vi "Teleop.vi"(10 "Match Info out":T2={"Autonomous Elapsed Seconds"=0.0, "TeleOp Elapsed Seconds"=0.0, "Disabled Elapsed Seconds"=0.0, "Visited Autonomous"=FALSE, "Visited TeleOp"=FALSE, "Visited Disabled"=FALSE, "Autonomous Settings"={"Autonomous Style"=enum."Independent", "VI Refnum"=refnum}}, 11 "Call Context":T3) -> ()   [LabVIEW 2015]
doc: "This VI is called for each TeleOp packet received from the DS where the robot is not disabled. It is often used to read from the joysticks and update I/O or to update setpoints for timed control loops. It should complete and return within 20 milliseconds or it may miss DS packets."
uses:
  Robot Global Data.vi
  <vilib>/Rock Robotics/WPI/RobotDrive/WPI_RobotDriveMecanumDrive_Cartesian.vi
  <vilib>/addons/control/pid/NI_PID_pid.lvlib
  <vilib>/addons/control/pid/pid.llb/PID (DBL).vi
  <vilib>/Rock Robotics/WPI/DriverStation/WPI_DriverStationDerivedRobotMode.ctl
  <vilib>/Rock Robotics/WPI/DriverStation/WPI_DriverStationMatch Info.ctl
panel:
  out "Gyro":T1(graph)
  out "Rotation Input":dbl(graph)
  out "Numeric 1":dbl(slide) scale=0.0..100.0
  out "Boolean 2":bool
  out "Boolean 1":bool
  in  "Match Info":T2={"Autonomous Elapsed Seconds"=0.0, "TeleOp Elapsed Seconds"=0.0, "Disabled Elapsed Seconds"=0.0, "Visited Autonomous"=FALSE, "Visited TeleOp"=FALSE, "Visited Disabled"=FALSE, "Autonomous Settings"={"Autonomous Style"=enum."Independent", "VI Refnum"=refnum}}
  in  "Call Context 2":T3
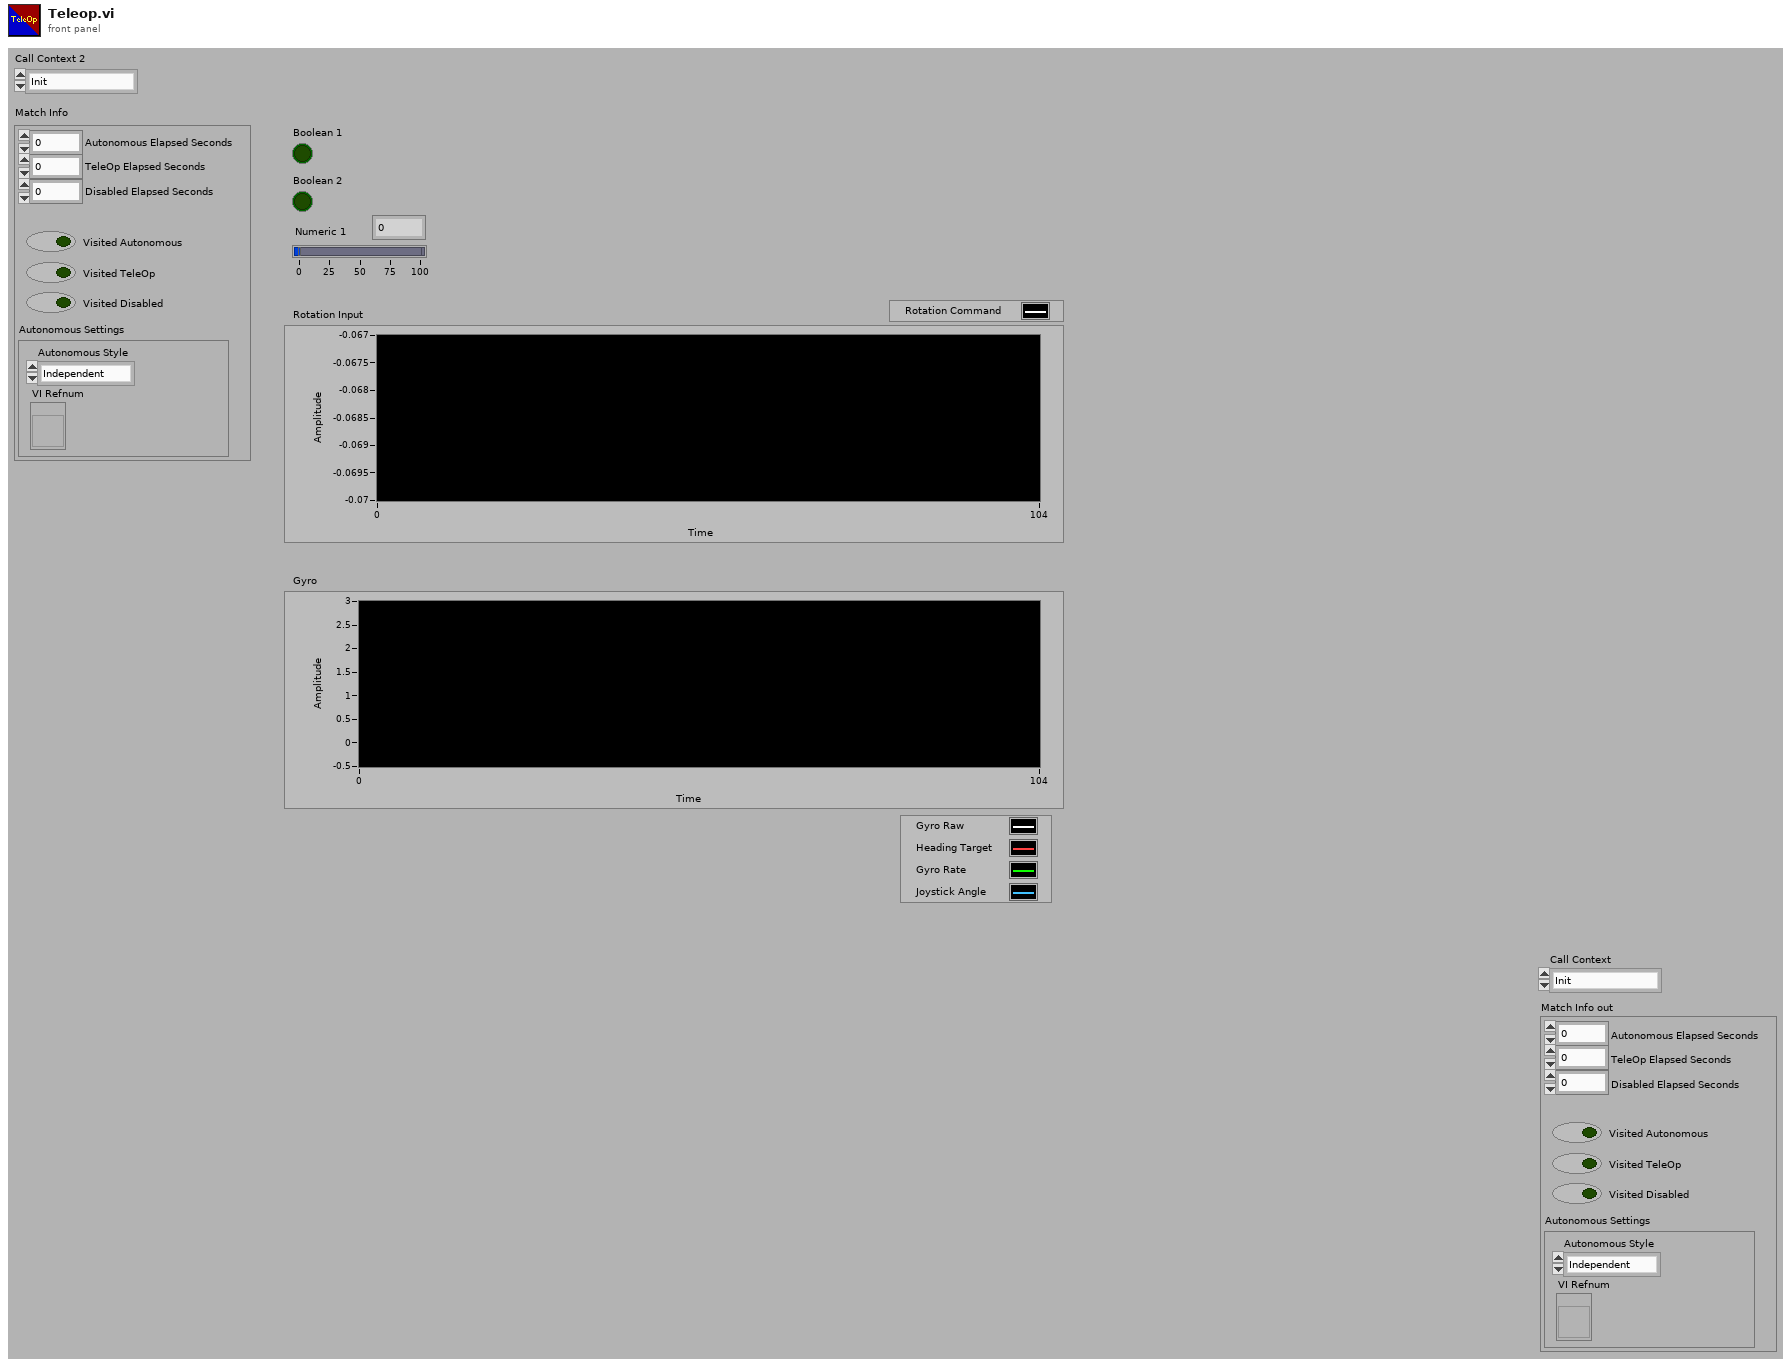
[diagram p1: front panel]
types:
  T1 = cluster{"Angle":dbl, "Heading":dbl, "Angular Rate":dbl, dbl}
  T2 = typedef "WPI_DriverStationMatch Info.ctl" = cluster{"Autonomous Elapsed Seconds":dbl, "TeleOp Elapsed Seconds":dbl, "Disabled Elapsed Seconds":dbl, "Visited Autonomous":bool, "Visited TeleOp":bool, "Visited Disabled":bool, "Autonomous Settings":cluster{"Autonomous Style":enum16{"Iterative", "Independent"}, "VI Refnum":refnum<vi>}}
  T3 = typedef "WPI_DriverStationDerivedRobotMode.ctl" = enum16{"Init", "Execute", "Stop"}
  T4 = cluster{"proportional gain (Kc)":dbl, "integral time (Ti, min)":dbl, "derivative time (Td, min)":dbl}
  T5 = typedef "WPI_JoystickDevRef.ctl" = cluster{"Device":T6}
  T6 = typedef "WPI_JoystickDeviceEnum.ctl" = enum16{"USB 0", "USB 1", "USB 2", "USB 3", "USB 4", "USB 5"}
  T7 = cluster{"Button 1":bool, "Button 2":bool, "Button 3":bool, "Button 4":bool, "Button 5":bool, "Button 6":bool, "Button 7":bool, "Button 8":bool, "Button 9":bool, "Button 10":bool, "Button 11":bool, "Button 12":bool}
  T8 = cluster{"axis 1 (x)":dbl, "axis 2 (y)":dbl, "axis 3 (throttle)":dbl, "axis 4":dbl, "axis 5":dbl, "axis 6":dbl}
  T9 = typedef "WPI_GyroDevRef.ctl" = cluster{"DevStatus":errorcluster, "Analog Channel":T10, "Offset":dbl, "Gain (VoltsPerDegree/Second)":dbl}
  T10 = typedef "FPGA_AIChannel.ctl" = enum8{"AI 0", "AI 1", "AI 2", "AI 3", "AI MXP 0", "AI MXP 1", "AI MXP 2", "AI MXP 3", "Invalid"}
  T11 = enum16{"CW_Fast", "CW_Slow", "CCW_Fast", "CCW_Slow", "Straight", "WaitingForStraight", "Rotate_Move"}
  T12 = typedef "WPI_RobotDriveDevRef.ctl" = cluster{"DevStatus":errorcluster, "Motors[]":T13[], "Square Inputs":bool, "Max Output":dbl}
  T13 = typedef "WPI_MotorControlDeviceRef.ctl" = cluster{"DeviceStatus":errorcluster, "Type":T14, "PWM":cluster{"PWM Channel":T15, "DeadBand":T16}, "CAN":cluster{"Device Number":u8, "Control Mode":T17, "Semaphore":T18, "Max Vout":dbl, "TalonSRX Control Mode":T19}, "Invert":bool, "TransformRef":T20, "InvTransformRef":T20}
  T14 = typedef "WPI_MotorControlType.ctl" = enum16{"PWM", "CAN", "CANTalonSRX"}
  T15 = typedef "FPGA_DIOPWMChannel.ctl" = enum8{"PWM 0", "PWM 1", "PWM 2", "PWM 3", "PWM 4", "PWM 5", "PWM 6", "PWM 7", "PWM 8", "PWM 9", "PWM MXP 0", "PWM MXP 1", "PWM MXP 2", "PWM MXP 3", "PWM MXP 4", "PWM MXP 5", "PWM MXP 6", "PWM MXP 7", "PWM MXP 8", "PWM MXP 9", "Invalid"}
  T16 = typedef "WPI_PWMDeadband.ctl" = cluster{"Name":string, "maxPositivePwm":i32, "minPositivePwm":i32, "centerPwm":i32, "maxNegativePwm":i32, "minNegativePwm":i32, "angularRange":u16}
  T17 = typedef "WPI_CANJaguar_ControlMode.ctl" = enum8{"Percent VBus", "Current", "Speed", "Position", "Voltage"}
  T18 = typedef "Semaphore RefNum" = refnum<k1>
  T19 = typedef "WPI_CANTalonSRX_APIControlMode.ctl" = enum8{"Percent VBus", "Speed", "Position", "Slave", "Unchanged / Invalid"}
  T20 = typedef "WPI_PWMTransform_ConPane.ctl" = refnum<vi>
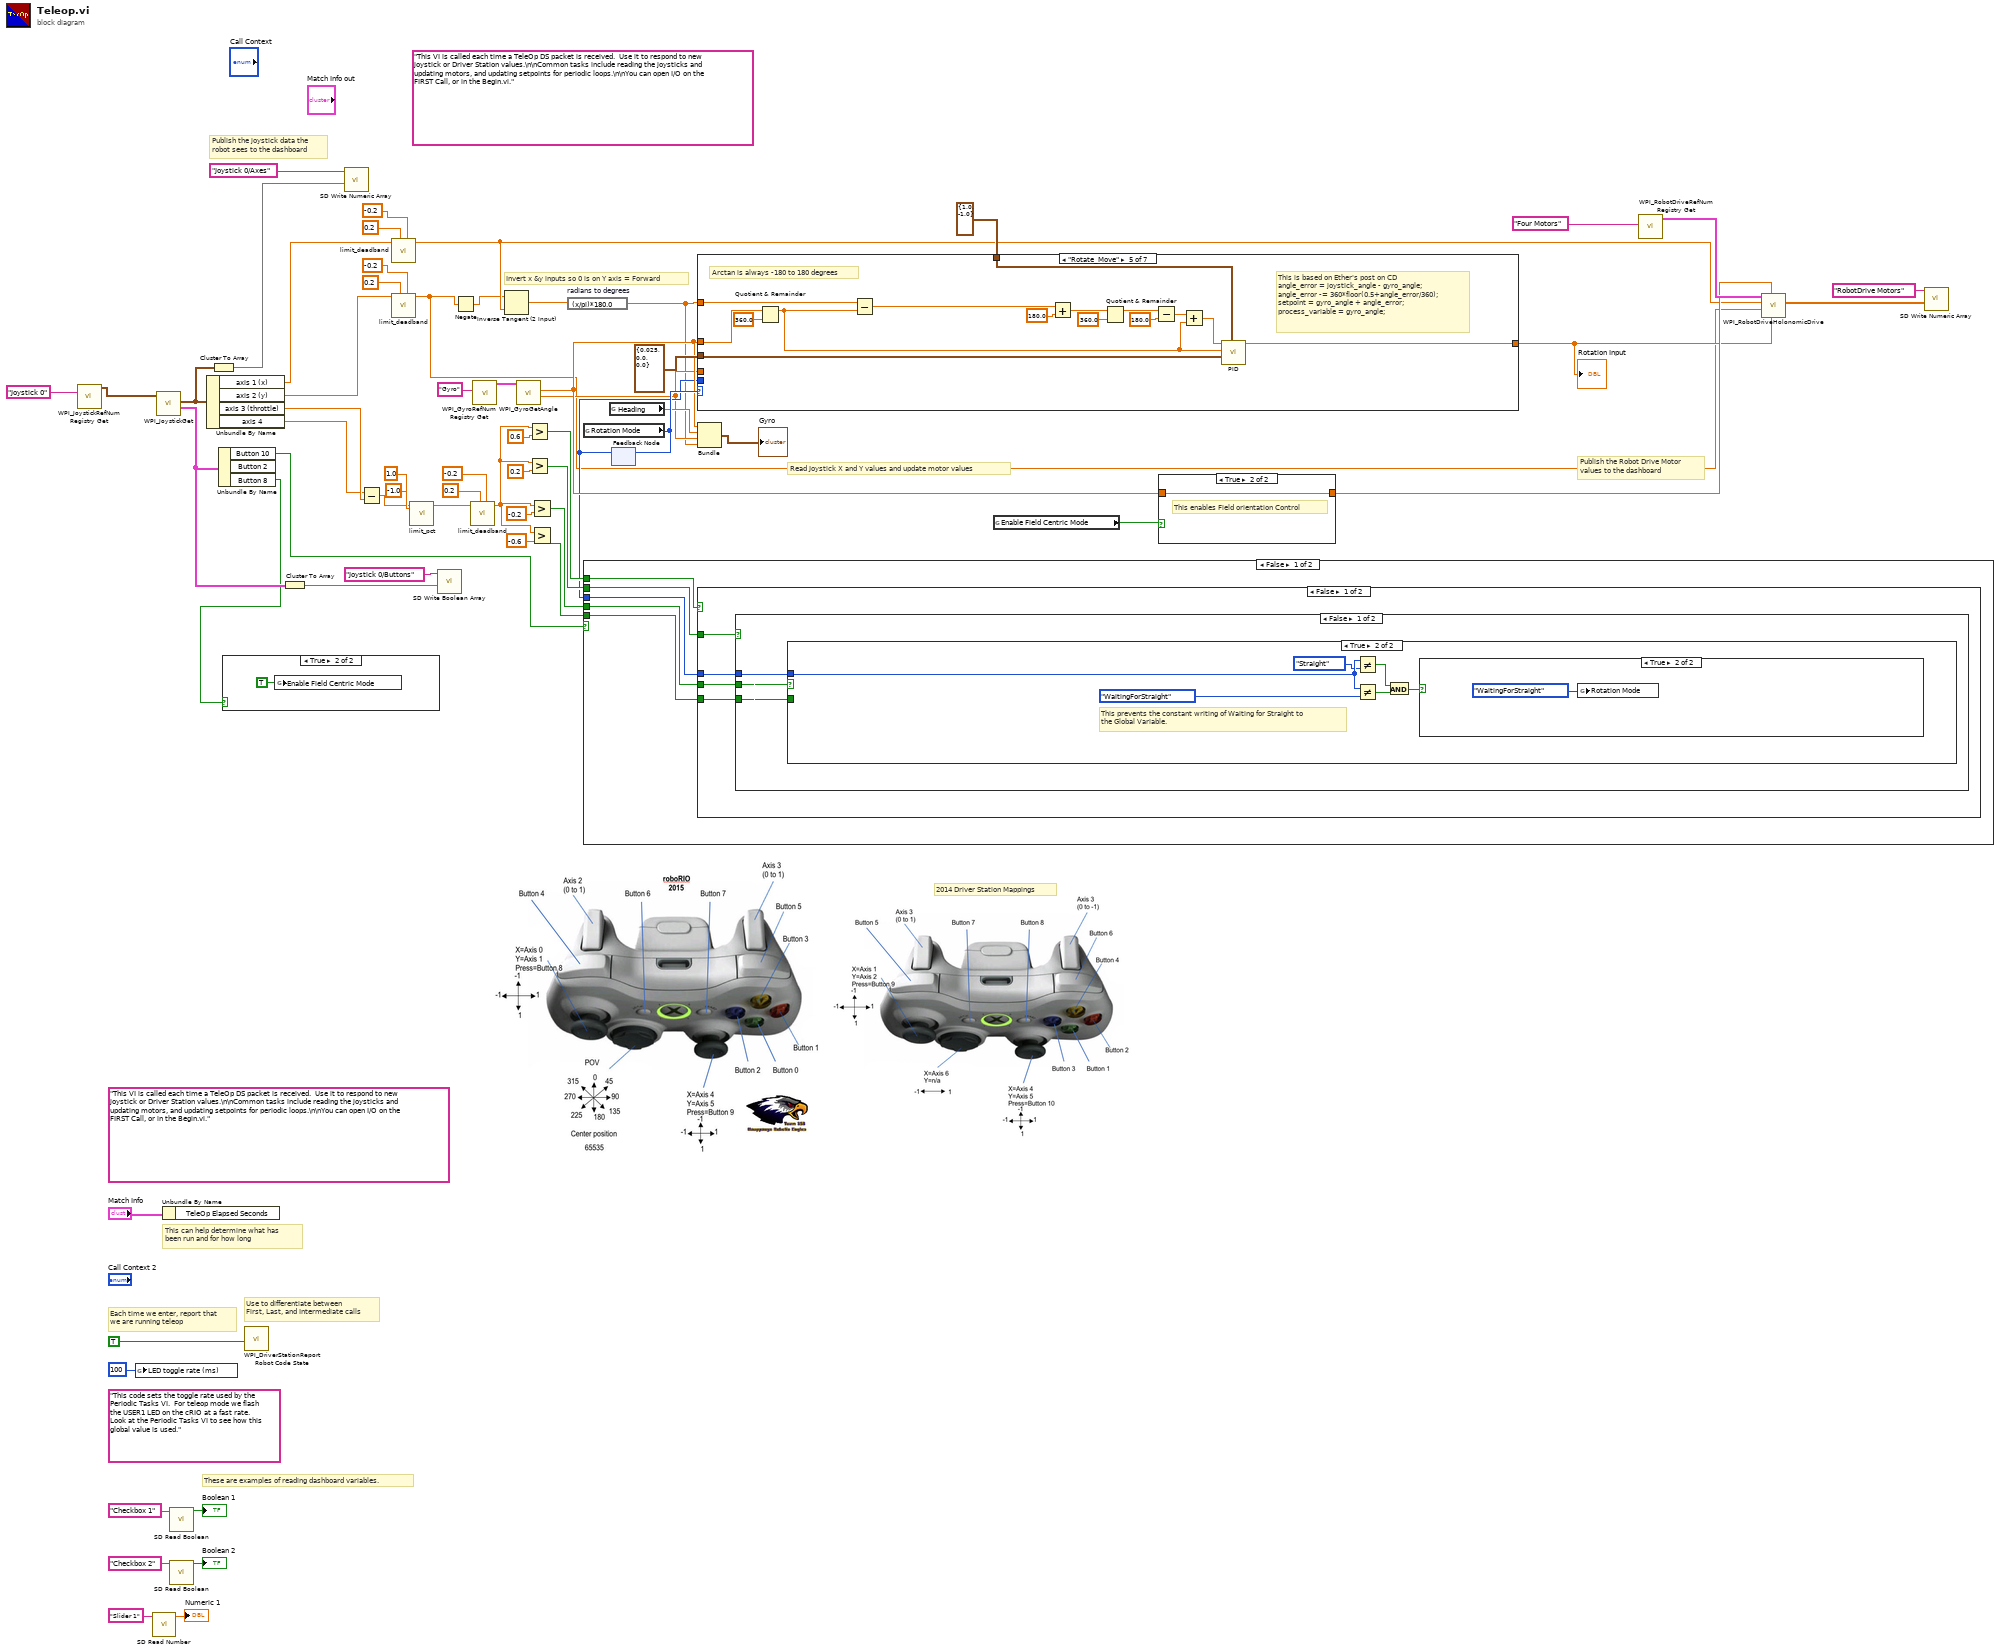
[diagram p0: block diagram]
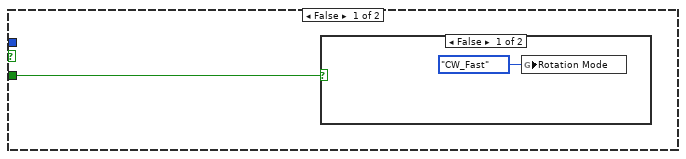
[diagram p3: hidden frame]
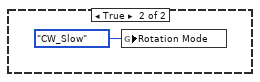
[diagram p4: hidden frame]
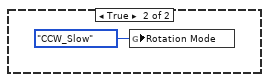
[diagram p6: hidden frame]
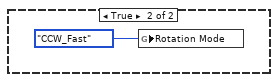
[diagram p7: hidden frame]
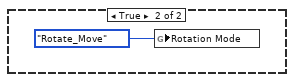
[diagram p8: hidden frame]
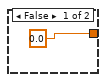
[diagram p9: hidden frame]
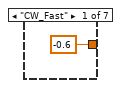
[diagram p10: hidden frame]
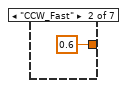
[diagram p11: hidden frame]
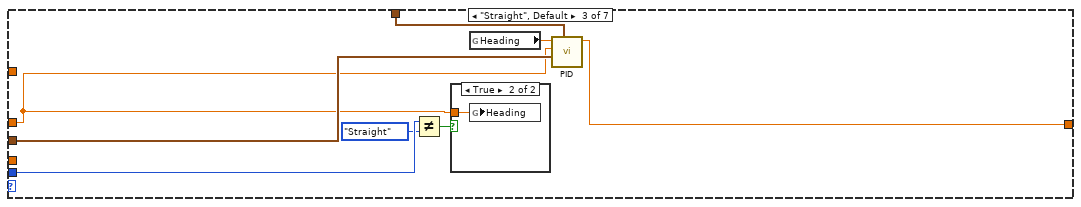
[diagram p12: hidden frame]
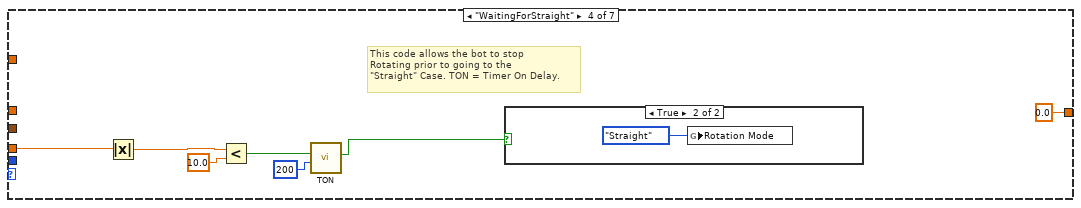
[diagram p14: hidden frame]
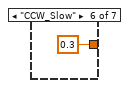
[diagram p16: hidden frame]
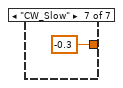
[diagram p17: hidden frame]
diagram:
  (unwired) "This code sets the toggle rate used by the Periodic Tasks VI.  For teleop mode we flash the USER1 LED on the cRIO at a fast rate.  Look at the Periodic Tasks VI to see how this global value is used."
  (unwired) "This VI is called each time a TeleOp DS packet is received.  Use it to respond to new joystick or Driver Station values.\n\nCommon tasks include reading the joysticks and updating motors, and updating setpoints for periodic loops.\n\nYou can open I/O on the FIRST Call, or in the Begin.vi."
  (unwired) "This VI is called each time a TeleOp DS packet is received.  Use it to respond to new joystick or Driver Station values.\n\nCommon tasks include reading the joysticks and updating motors, and updating setpoints for periodic loops.\n\nYou can open I/O on the FIRST Call, or in the Begin.vi."
  # "Invert x &y inputs so 0 is on Y axis = Forward"
  # "2014 Driver Station Mappings"
  # "These are examples of reading dashboard variables."
  # "Publish the Robot Drive Motor\nvalues to the dashboard"
  # "Publish the joystick data the\nrobot sees to the dashboard"
  # "Each time we enter, report that\nwe are running teleop"
  # "Use to differentiate between\nFirst, Last, and Intermediate calls"
  # "This can help determine what has\nbeen run and for how long"
  # "Read Joystick X and Y values and update motor values"
  n1 = call <vilib>:"WPI_JoystickRefNum Registry Get.vi"("refnum name"="Joystick 0") -> ("JoystickDevRef"=w60:T5)  [unwired: 1 in, 9 out]
  n2 = global write "Robot Global Data.vi" "LED toggle rate (ms)"(u32 100 ("LED ms toggle rate")) -> ()
  n3 = call <vilib>:"SD Read Number.vi"("Name"="Slider 1" ("refnum name")) -> ("Numeric"=→"Numeric 1":dbl)  [unwired: 8 in, 2 out]
  n4 = call <vilib>:"WPI_JoystickGet.vi"("JoystickDevRef"=w60) -> ("Buttons"=w24:T7, "Axes"=w55:T8)  [unwired: 1 in, 4 out]
  n5 = Unbundle By Name("Match Info") -> ()  [unwired: 1 out]
  n6 = call <vilib>:"SD Read Boolean.vi"("Name"="Checkbox 1" ("refnum name")) -> ("Boolean"=→"Boolean 1":bool)  [unwired: 8 in, 2 out]
  n7 = call <vilib>:"SD Read Boolean.vi"("Name"="Checkbox 2" ("refnum name")) -> ("Boolean"=→"Boolean 2":bool)  [unwired: 8 in, 2 out]
  n8 = Unbundle By Name(w55) -> ("axis 1 (x)"=w21:dbl, "axis 2 (y)"=w6:dbl, "axis 3 (throttle)"=w10:dbl, "axis 4"=w9:dbl)
  n9 = Cluster To Array(cluster=w55) -> (array=w54:dbl[])
  n10 = Unbundle By Name(w24) -> ("Button 10"=w22:bool, "Button 8"=w8:bool)  [unwired: 1 out]
  n11 = case shown="True" w8 {
    frame False {
    }
    frame True {
      n12 = global write "Robot Global Data.vi" "Enable Field Centric Mode"(TRUE ("Enable Field Centric Mode")) -> ()
    }
  }
  n13 = call <vilib>:"WPI_DriverStationReport Robot Code State.vi"("TeleOp"=TRUE ("Autonomous")) -> ()  [unwired: 10 in, 1 out]
  n14 = Cluster To Array(cluster=w24) -> (array=w57:bool[])
  n15 = call <vilib>:"SD Write Numeric Array.vi"("Numeric Array"=w54, "Name"="Joystick 0/Axes") -> ()  [unwired: 8 in, 2 out]
  n16 = Subtract(x=w9, y=w10) -> (x-y=w11:dbl)
  n17 = call "limit_deadband.vi"("lower limit"=-0.2, "upper limit"=0.2, "Val"=w21) -> ("Val Out"=w4:dbl)  [unwired: 8 in]
  n18 = call "limit_deadband.vi"("lower limit"=-0.2, "upper limit"=0.2, "Val"=w6) -> ("Val Out"=w5:dbl)  [unwired: 8 in]
  n19 = call "limit_pct.vi"("upper limit"=1.0, "lower limit"=-1.0, "PCT"=w11) -> ("PCT Out"=w34:dbl)  [unwired: 8 in]
  n20 = call <vilib>:"SD Write Boolean Array.vi"("Boolean Array"=w57, "Name"="Joystick 0/Buttons") -> ()  [unwired: 8 in, 2 out]
  n21 = Negate(x=w5) -> (-x=w3:dbl)
  n22 = call "limit_deadband.vi"("lower limit"=-0.2, "upper limit"=0.2, "Val"=w34) -> ("Val Out"=w27:dbl)  [unwired: 8 in]
  n23 = call <vilib>:"WPI_GyroRefNum Registry Get.vi"("refnum name"="Gyro") -> ("GyroDevRef"=w44:T9)  [unwired: 9 in, 1 out]
  n24 = Inverse Tangent (2 Input)(1:w4, 2:w3) -> (0:w1:dbl)
  n25 = call <vilib>:"WPI_GyroGetAngle.vi"("GyroDevRef"=w44) -> ("Angular Rate"=w13:dbl, "Angle"=w16:dbl)  [unwired: 7 in, 2 out]
  n26 = Greater?(x=w27, y=0.6 ("x")) -> (0:w33:bool)
  n27 = Greater?(x=w27, y=0.2 ("x")) -> (0:w32:bool)
  n28 = Greater?(x=w27, y=-0.2) -> (0:w28:bool)
  n29 = Greater?(x=w27, y=-0.6) -> (0:w25:bool)
  n30 = expression code="(x/pi)*180.0" "radians to degrees"(w1) -> (w2:dbl)
  n31 = global read "Robot Global Data.vi" "Rotation Mode"() -> (w18:T11)
  n32 = global read "Robot Global Data.vi" "Heading"() -> (w15:dbl)
  n33 = feedback #1() -> (w14:T11)  [unwired: 1 in]
  n34 = case shown="False" w22 {
    tunnel: w33 -> [w70 _]
    tunnel: w32 -> [w69 _]
    tunnel: w28 -> [w68 _]
    tunnel: w25 -> [w67 _]
    tunnel: w14 -> [w66 _]
    frame False {
      n35 = case shown="False" w70 {
        tunnel: w69 -> [w74 _]
        tunnel: w68 -> [w73 _]
        tunnel: w67 -> [w72 _]
        tunnel: w66 -> [w71 _]
        frame False {
          n36 = case shown="False" w74 {
            tunnel: w73 -> [w77 _]
            tunnel: w72 -> [w76 _]
            tunnel: w71 -> [w75 _]
            frame False {
              n37 = case shown="True" w77 {
                tunnel: w76 -> [w78 _]
                tunnel: w75 -> [_ w86]
                frame False {
                  n38 = case shown="False" w78 {
                    frame False {
                      n39 = global write "Robot Global Data.vi" "Rotation Mode"(T11."CW_Fast" ("Rotation Mode")) -> ()
                    }
                    frame True {
                      n40 = global write "Robot Global Data.vi" "Rotation Mode"(T11."CW_Slow" ("Rotation Mode")) -> ()
                    }
                  }
                }
                frame True {
                  # "This prevents the constant writing of Waiting for Straight to \nthe Global Variable."
                  n41 = Not Equal?(x=w86, y=T11."Straight") -> (x != y?=w82:bool)
                  n42 = Not Equal?(x=w86, y=T11."WaitingForStraight") -> (x != y?=w81:bool)
                  n43 = And(x=w82, y=w81) -> (x .and. y?=w83:bool)
                  n44 = case shown="True" w83 {
                    frame False {
                    }
                    frame True {
                      n45 = global write "Robot Global Data.vi" "Rotation Mode"(T11."WaitingForStraight" ("Rotation Mode")) -> ()
                    }
                  }
                }
              }
            }
            frame True {
              n46 = global write "Robot Global Data.vi" "Rotation Mode"(T11."CCW_Slow" ("Rotation Mode")) -> ()
            }
          }
        }
        frame True {
          n47 = global write "Robot Global Data.vi" "Rotation Mode"(T11."CCW_Fast" ("Rotation Mode")) -> ()
        }
      }
    }
    frame True {
      n48 = global write "Robot Global Data.vi" "Rotation Mode"(T11."Rotate_Move" ("Rotation Mode")) -> ()
    }
  }
  n49 = feedback-in #1(w18) -> ()
  n50 = case shown="\"Rotate_Move\"" w18 {
    tunnel: [-0.6 ("Rotation") 0.6 ("Rotation") w94 0.0 ("Rotation") w124 0.3 ("Rotation") -0.3 ("Rotation")] -> w17
    tunnel: w16 -> [_ _ w93 _ w111 _ _]
    tunnel: w13 -> [_ _ _ w103 _ _ _]
    tunnel: T4 {"proportional gain (Kc)"=0.025, "integral time (Ti, min)"=0.0, "derivative time (Td, min)"=0.0} ("PID gains") -> [_ _ w95 _ w123 _ _]
    tunnel: w2 -> [_ _ _ _ w117 _ _]
    tunnel: cluster{"output high":dbl, "output low":dbl} {"output high"=1.0, "output low"=-1.0} ("output range") -> [_ _ w96 _ w120 _ _]
    tunnel: w14 -> [_ _ w100 _ _ _ _]
    frame "CW_Fast" {
    }
    frame "CCW_Fast" {
    }
    frame "Straight", Default {
      n51 = Not Equal?(x=w100, y=T11."Straight" ("Rotation Mode")) -> (x != y?=w97:bool)
      n52 = case shown="True" w97 {
        tunnel: w93 -> [_ w101]
        frame False {
        }
        frame True {
          n53 = global write "Robot Global Data.vi" "Heading"(w101) -> ()
        }
      }
      n54 = global read "Robot Global Data.vi" "Heading"() -> (w98:dbl)
      n55 = call-poly <vilib>:"PID.vi"("output range"=w96, "PID gains"=w95, "process variable"=w93, "setpoint"=w98) -> ("output"=w94:dbl)  [unwired: 6 in, 1 out]
    }
    frame "WaitingForStraight" {
      # "This code allows the bot to stop \nRotating prior to going to the \n\"Straight\" Case. TON = Timer On Delay."
      n56 = Absolute Value(x=w103) -> (abs(x)=w102:dbl)
      n57 = Less?(x=w102, y=10.0) -> (x < y?=w105:bool)
      n58 = call "TON.vi"("Delay (ms)"=u32 200, "Input"=w105) -> ("Output"=w106:bool)  [unwired: 9 in]
      n59 = case shown="True" w106 {
        frame False {
        }
        frame True {
          n60 = global write "Robot Global Data.vi" "Rotation Mode"(T11."Straight" ("Rotation Mode")) -> ()
        }
      }
    }
    frame "Rotate_Move" {
      # "Arctan is always -180 to 180 degrees"
      # "This is based on Ether's post on CD\nangle_error = joystick_angle - gyro_angle;\nangle_error -= 360*floor(0.5+angle_error/360);\nsetpoint = gyro_angle + angle_error;\nprocess_variable = gyro_angle;"
      n61 = Quotient & Remainder(x=w111, y=360.0) -> (x-y*floor(x/y)=w110:dbl)  [unwired: 1 out]
      n62 = Subtract(x=w117, y=w110) -> (x-y=w119:dbl)
      n63 = Add(x=w119, y=180.0) -> (x+y=w116:dbl)
      n64 = Quotient & Remainder(x=w116, y=360.0) -> (x-y*floor(x/y)=w115:dbl)  [unwired: 1 out]
      n65 = Subtract(x=w115, y=180.0) -> (x-y=w113:dbl)
      n66 = Add(x=w113, y=w110) -> (x+y=w112:dbl)
      n67 = call-poly <vilib>:"PID.vi"("output range"=w120, "PID gains"=w123, "process variable"=w110, "setpoint"=w112) -> ("output"=w124:dbl)  [unwired: 6 in, 1 out]
    }
    frame "CCW_Slow" {
    }
    frame "CW_Slow" {
    }
  }
  "Rotation Input" <- w17
  n68 = Bundle("Angle"=w16, "Heading"=w15, "Angular Rate"=w13, w2) -> (→"Gyro":T1)  [unwired: 1 in]
  n69 = global read "Robot Global Data.vi" "Enable Field Centric Mode"() -> (w7:bool)
  n70 = case shown="True" w7 {
    tunnel: w16 -> [_ w128]
    tunnel: [0.0 ("Angle") w128] -> w23
    frame False {
    }
    frame True {
      # "This enables Field orientation Control"
    }
  }
  n71 = call <vilib>:"WPI_RobotDriveRefNum Registry Get.vi"("refnum name"="Four Motors") -> ("RobotDriveDevRef"=w62:T12)  [unwired: 1 in, 9 out]
  n72 = call-poly <vilib>:"WPI_RobotDriveHolonomicDrive.vi"("Rotation"=w17, "Gyro Angle"=w23, "Y"=w5, "X"=w4, "RobotDriveDevRef"=w62) -> ("Motor Values"=w51:dbl[])  [unwired: 4 in, 2 out]
  n73 = call <vilib>:"SD Write Numeric Array.vi"("Numeric Array"=w51, "Name"="RobotDrive Motors") -> ()  [unwired: 8 in, 2 out]
